vi "Cleanup.vi"(8 "error in (no error)":errorcluster, 11 "GVIWebProcessorApp in":refnum<class "GVIWebProcessorApp.lvclass">) -> (0 "error out":errorcluster)   [LabVIEW 2020, in "PicoG-Processor.lvlib" / "GVIWebProcessorApp.lvclass"]
uses:
  GVIWebProcessorApp.lvclass
  GVIWebProcessorApp.lvclass/GVIWebProcessorApp.ctl
  <vilib>/IlluminatedG/IG OOPanel/OOPanel/ArrayManager/ArrayManager.lvclass
  WebProjectWatcher/WebProjectWatcher.lvclass
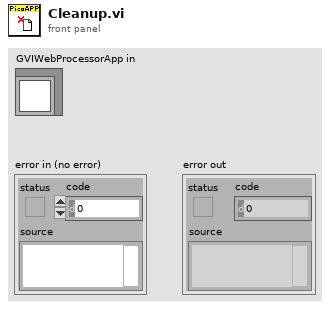
[diagram p1: front panel]
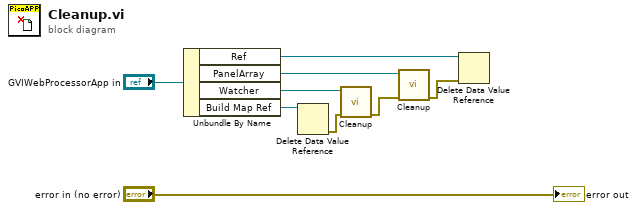
[diagram p0: block diagram]
diagram:
  n1 = Unbundle By Name("GVIWebProcessorApp in") -> ("Ref"=w7:refnum<data-value>, "PanelArray"=w5:refnum<class "ArrayManager.lvclass">, "Watcher"=w4:refnum<class "WebProjectWatcher.lvclass">, "Build Map Ref"=w2:refnum<data-value>)
  n2 = Delete Data Value Reference(data value reference=w2) -> (error out=w1:errorcluster)  [unwired: 1 in, 1 out]
  n3 = call <vilib>:"Cleanup.vi"("error in (no error)"=w1, "WebProjectWatcher in"=w4) -> ("error out"=w3:errorcluster)  [unwired: 9 in]
  n4 = call <vilib>:"Cleanup.vi"("error in (no error)"=w3, "PanelArray in"=w5) -> ("error out"=w6:errorcluster)  [unwired: 7 in, 2 out]
  n5 = Delete Data Value Reference(data value reference=w7, error in=w6) -> ()  [unwired: 2 out]
  "error out" <- "error in (no error)"
